vi "WriteSettingsAndActuators.vi"(10 "SettingsActuators":T1, 11 "Refnum in":refnum<k20>) -> (0 "error out":errorcluster)   [LabVIEW 2019]
uses:
  Settings_Actuators.ctl
  <vilib>/Utility/error.llb/Error Cluster From Error Code.vi
  <vilib>/rvi/errors/niLvFpgaAdjustHostInterfaceError.vi
  <vilib>/rvi/interface/nirviReadWriteControl/nirviReadWriteControl.xnode
  NiFpgaLv.dll
  <vilib>/rvi/interface/Simulation/niFpgaSimulationCallBeginRW.vi
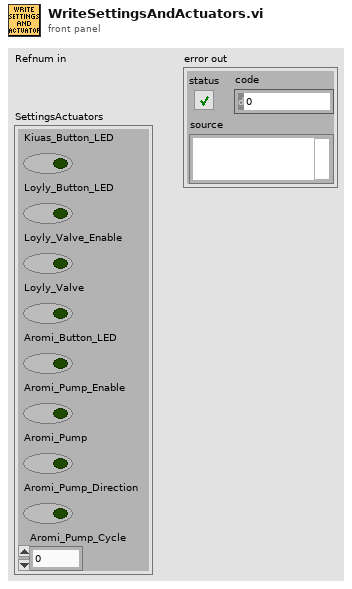
[diagram p1: front panel]
types:
  T1 = typedef "Settings_Actuators.ctl" = cluster{"Kiuas_Button_LED":bool, "Loyly_Button_LED":bool, "Loyly_Valve_Enable":bool, "Loyly_Valve":bool, "Aromi_Button_LED":bool, "Aromi_Pump_Enable":bool, "Aromi_Pump":bool, "Aromi_Pump_Direction":bool, "Aromi_Pump_Cycle":u32}
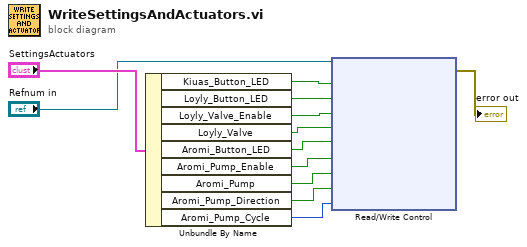
[diagram p0: block diagram]
diagram:
  n1 = Unbundle By Name("SettingsActuators") -> ("Kiuas_Button_LED"=w3:bool, "Loyly_Button_LED"=w4:bool, "Loyly_Valve_Enable"=w5:bool, "Loyly_Valve"=w6:bool, "Aromi_Button_LED"=w7:bool, "Aromi_Pump_Enable"=w8:bool, "Aromi_Pump"=w9:bool, "Aromi_Pump_Direction"=w10:bool, "Aromi_Pump_Cycle"=w11:u32)
  n2 = xnode "Read/Write Control"("FPGA VI Reference In"="Refnum in", "Kiuas LED"=w3, "Löyly LED"=w4, "Löyly Valve Enable"=w5, "Löyly Valve"=w6, "Aromi LED"=w7, "Aromi Pump Enable"=w8, "Aromi Pump"=w9, "Pump Direction"=w10, "Pump Cycle"=w11) -> ("error out"=→"error out":errorcluster)  [unwired: 1 in, 1 out]
